vi "vibrate_and_record.vi"(3 "SSH password":string, 4 "Transfer and Run Date Folder After Experiment":bool, 5 "SSH user name":string, 6 "Tags":string, 7 "Frames":i32, 8 "frequencies":dbl[](array[numeric]), 9 "PWM duty cycles":dbl[](array[numeric]), 10 "parameters":string[](array[string]), 11 "parameters headers":string[](array[string])) -> ()   [LabVIEW 2014]
uses:
  <vilib>/userdefined/High Color/IMAQdx.ctl
  <vilib>/Utility/file.llb/Write To Spreadsheet File (DBL).vi
  <vilib>/Utility/file.llb/Write To Spreadsheet File (string).vi
  <vilib>/Utility/file.llb/Read From Spreadsheet File (string).vi
  <vilib>/vision/driver/NI_Vision_Acquisition_Software.lvlib
panel:
  out "Error":string
  out "Save Directory":path
  out "Buffer Number Out":u32
  out "Image":T1(plugin-control)
  in  "stop":bool
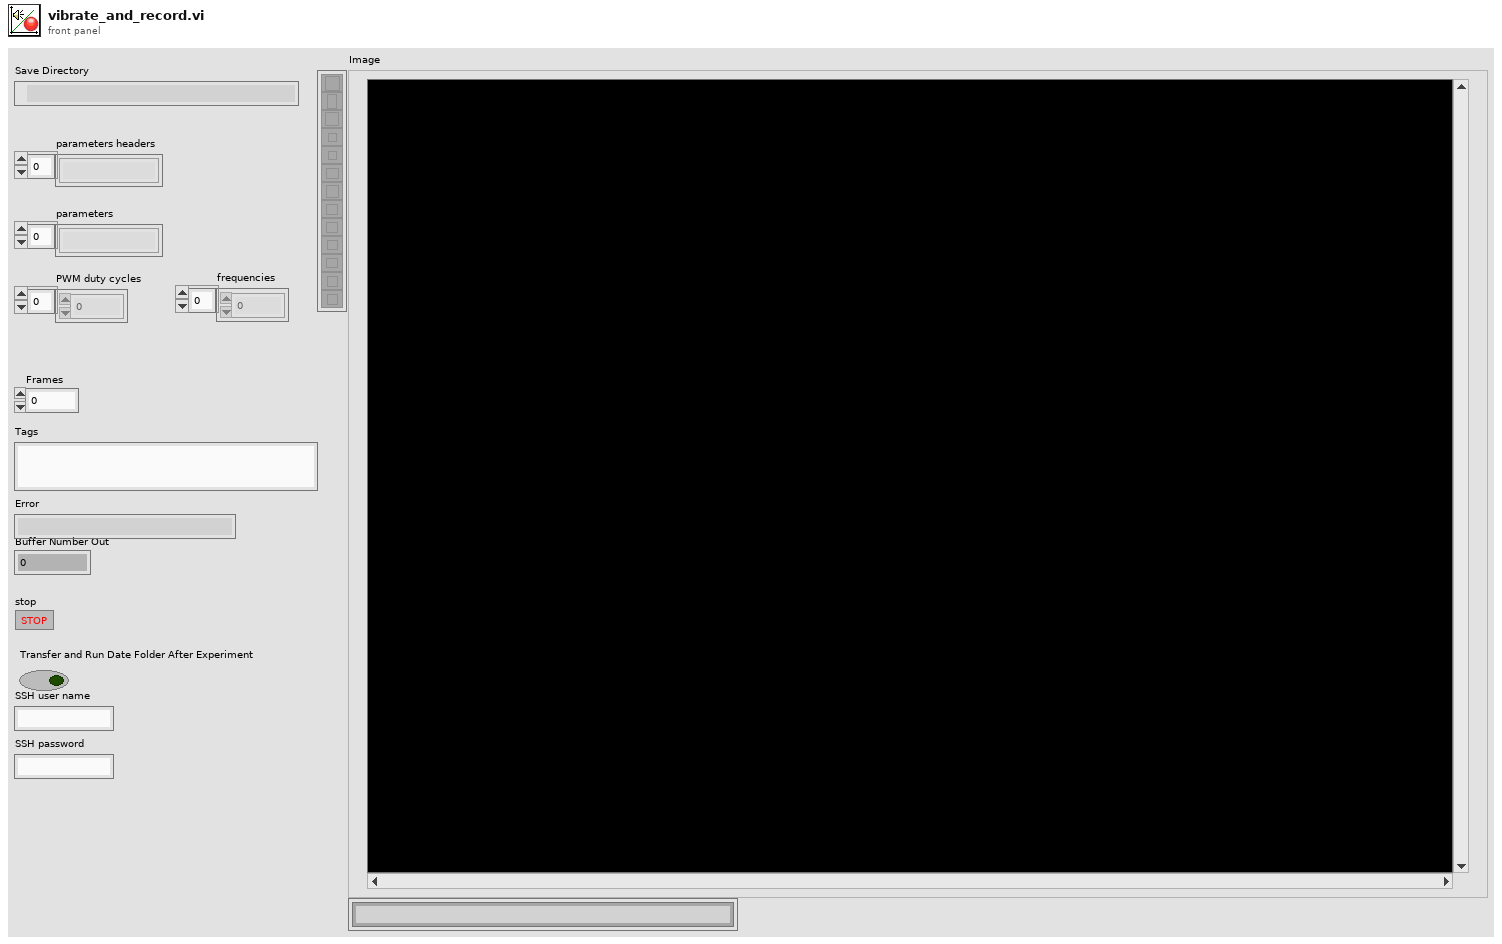
[diagram p1: front panel]
types:
  T1 = typedef "IMAQ Image.ctl" = refnum<image>
  T2 = typedef "IMAQdx.ctl" = refnum<k21>
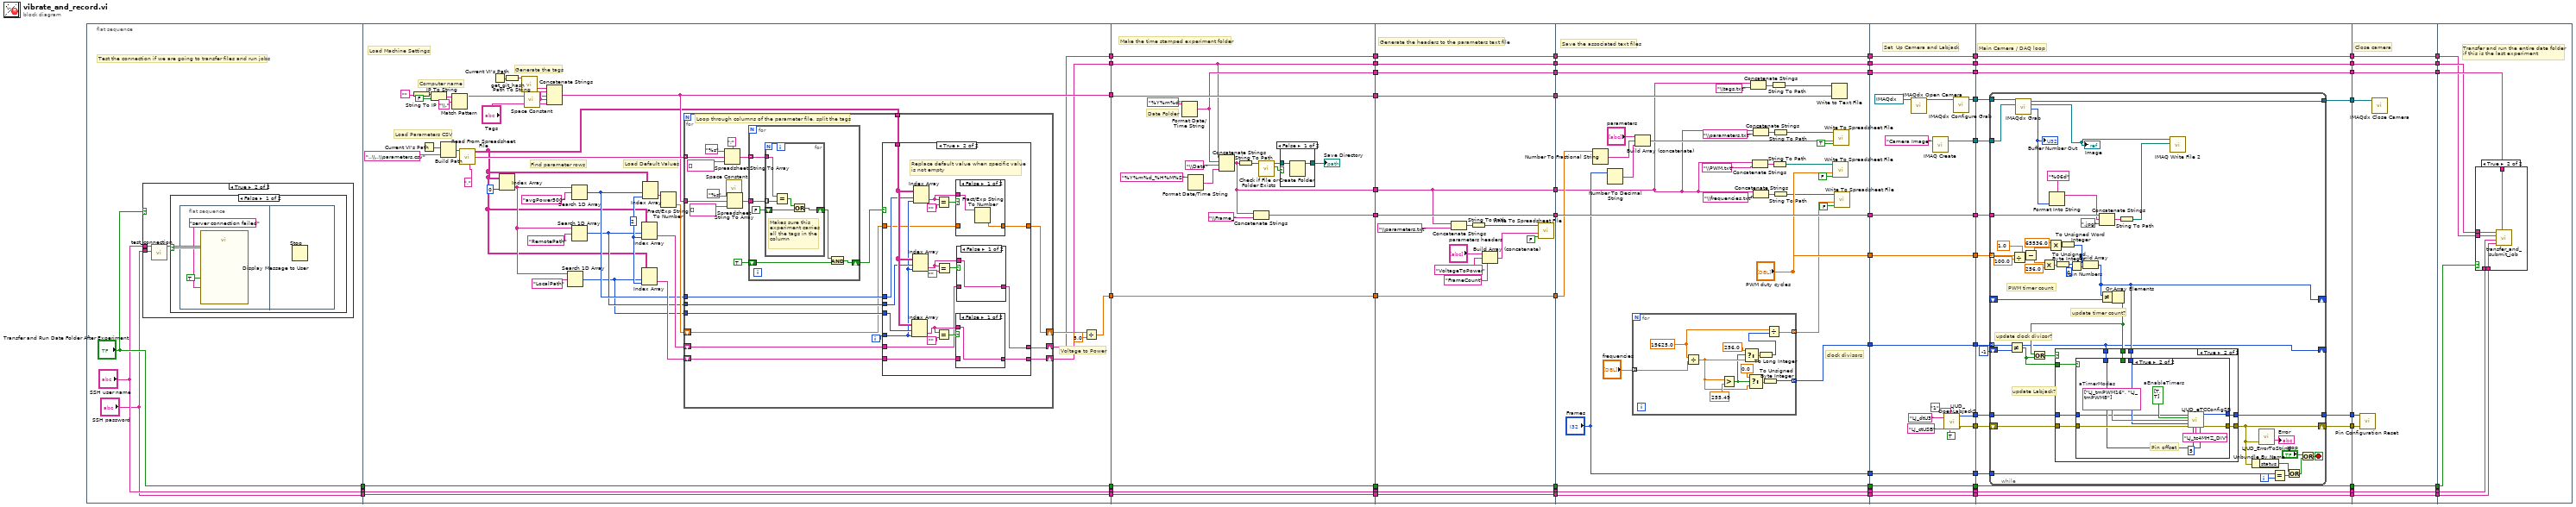
[diagram p0: block diagram]
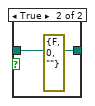
[diagram p8: hidden frame]
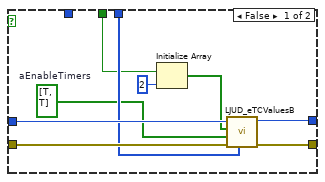
[diagram p10: hidden frame]
diagram:
  n1 = flat-sequence {
    tunnel: ["Transfer and Run Date Folder After Experiment"] -> w28
    tunnel: ["SSH user name"] -> w27
    tunnel: ["SSH password"] -> w26
    tunnel: [w108] -> w58
    tunnel: [w88] -> w57
    tunnel: [w78] -> w48
    tunnel: [w79] -> w47
    tunnel: w28 -> [w99]
    tunnel: w27 -> [w98]
    tunnel: w26 -> [w97]
    tunnel: [w99] -> w19
    tunnel: [w98] -> w12
    tunnel: [w97] -> w11
    tunnel: [w199] -> w42
    tunnel: [w198] -> w40
    tunnel: [w197] -> w38
    tunnel: [w196] -> w36
    tunnel: [w195] -> w34
    tunnel: [w194] -> w32
    tunnel: [w193] -> w30
    tunnel: w47 -> [w193]
    tunnel: w48 -> [w194]
    tunnel: w57 -> [w196]
    tunnel: w58 -> [w197]
    tunnel: [w183] -> w20
    tunnel: w19 -> [w183]
    tunnel: [w182] -> w13
    tunnel: w12 -> [w182]
    tunnel: w11 -> [w181]
    tunnel: [w181] -> w10
    tunnel: w42 -> [w220]
    tunnel: [w220] -> w41
    tunnel: w40 -> [w206]
    tunnel: [w206] -> w39
    tunnel: w38 -> [w219]
    tunnel: [w219] -> w37
    tunnel: w36 -> [w218]
    tunnel: [w218] -> w35
    tunnel: w34 -> [w217]
    tunnel: [w217] -> w33
    tunnel: w32 -> [w216]
    tunnel: [w216] -> w31
    tunnel: w30 -> [w215]
    tunnel: [w215] -> w29
    tunnel: [w205] -> w21
    tunnel: w20 -> [w205]
    tunnel: [w204] -> w14
    tunnel: w13 -> [w204]
    tunnel: w10 -> [w203]
    tunnel: [w203] -> w9
    tunnel: w41 -> [w252]
    tunnel: [w252] -> w63
    tunnel: ["PWM duty cycles"] -> w61
    tunnel: ["Frames"] -> w60
    tunnel: w39 -> [w224]
    tunnel: w37 -> [w235]
    tunnel: w35 -> [w230]
    tunnel: w33 -> [w241]
    tunnel: [w241] -> w53
    tunnel: [w240] -> w49
    tunnel: w31 -> [w240]
    tunnel: [w239] -> w43
    tunnel: w29 -> [w239]
    tunnel: [w233] -> w22
    tunnel: w21 -> [w233]
    tunnel: [w232] -> w15
    tunnel: w14 -> [w232]
    tunnel: w9 -> [w231]
    tunnel: [w231] -> w8
    tunnel: [w221] -> w4
    tunnel: w63 -> [w282]
    tunnel: [w284] -> w69
    tunnel: [w283] -> w68
    tunnel: [w282] -> w67
    tunnel: [w267] -> w65
    tunnel: [w268] -> w64
    tunnel: [w278] -> w62
    tunnel: w61 -> [w278]
    tunnel: w60 -> [w277]
    tunnel: [w277] -> w59
    tunnel: [w275] -> w54
    tunnel: w53 -> [w275]
    tunnel: [w274] -> w50
    tunnel: w49 -> [w274]
    tunnel: [w273] -> w44
    tunnel: w43 -> [w273]
    tunnel: [w272] -> w23
    tunnel: w22 -> [w272]
    tunnel: [w271] -> w16
    tunnel: w15 -> [w271]
    tunnel: w8 -> [w270]
    tunnel: [w270] -> w7
    tunnel: w4 -> [w269]
    tunnel: [w269] -> w3
    tunnel: w69 -> [w305]
    tunnel: w68 -> [w304]
    tunnel: w67 -> [w303]
    tunnel: [w302] -> w66
    tunnel: w65 -> [w301]
    tunnel: w64 -> [w300]
    tunnel: w62 -> [w299]
    tunnel: w59 -> [w298]
    tunnel: [w297] -> w55
    tunnel: w54 -> [w297]
    tunnel: [w296] -> w51
    tunnel: w50 -> [w296]
    tunnel: [w295] -> w45
    tunnel: w44 -> [w295]
    tunnel: [w294] -> w24
    tunnel: w23 -> [w294]
    tunnel: [w293] -> w17
    tunnel: w16 -> [w293]
    tunnel: w7 -> [w292]
    tunnel: [w292] -> w6
    tunnel: w3 -> [w289]
    tunnel: [w291] -> w2
    tunnel: [w290] -> w1
    tunnel: w66 -> [w387]
    tunnel: [w386] -> w56
    tunnel: w55 -> [w386]
    tunnel: [w385] -> w52
    tunnel: w51 -> [w385]
    tunnel: [w384] -> w46
    tunnel: w45 -> [w384]
    tunnel: [w383] -> w25
    tunnel: w24 -> [w383]
    tunnel: [w382] -> w18
    tunnel: w17 -> [w382]
    tunnel: w6 -> [w381]
    tunnel: [w381] -> w5
    tunnel: w2 -> [w380]
    tunnel: w1 -> [w379]
    tunnel: w56 -> [w393]
    tunnel: w52 -> [w392]
    tunnel: w46 -> [w391]
    tunnel: w25 -> [w390]
    tunnel: w18 -> [w389]
    tunnel: w5 -> [w388]
    frame #0 {
      # "Test the connection if we are going to transfer files and run jobs"
      n2 = case shown="True" "Transfer and Run Date Folder After Experiment" {
        tunnel: "SSH password" -> [_ w75]
        tunnel: "SSH user name" -> [_ w73]
        frame False {
        }
        frame True {
          n3 = call "test_connection.vi"("Username"=w73, "Password"=w75) -> ("Connection Successful"=w74:bool)  [unwired: 7 in]
          n4 = case shown="False" w74 {
            frame False {
              n5 = flat-sequence {
                frame #0 {
                  n6 = call "Display Message to User"("Enable"=TRUE, "Message"="server connection failed") -> ()  [unwired: 8 in, 2 out]
                }
                frame #1 {
                  n7 = Stop() -> ()  [unwired: 1 in]
                }
              }
            }
            frame True {
            }
          }
        }
      }
    }
    frame #1 {
      w90 = 2
      # "Generate the tags"
      # "Find parameter rows"
      # "Load Default Values"
      # "Voltage to Power"
      # "Load Parameters CSV"
      # "Computer name"
      # "Load Machine Settings"
      n8 = String To IP(1:"") -> (0:w116:u32)
      n9 = Current VI's Path() -> (path=w111:path)
      n10 = IP To String(1:FALSE, 2:w116) -> (0:w113:string)
      n11 = Build Path(base path=w111, name or relative path="..\\..\\parameters.csv") -> (appended path=w101:path)
      n12 = Match Pattern(string=w113, regular expression="\\.") -> (before substring=w91:string)  [unwired: 1 in, 3 out]
      n13 = call-poly <vilib>:"Read From Spreadsheet File.vi"("delimiter (\\t)"=",", "file path (dialog if empty)"=w101) -> ("first row"=w89:string[], "all rows"=w81:string[][])  [unwired: 5 in, 3 out]
      n14 = Current VI's Path() -> (path=w94:path)
      n15 = Index Array(array=w81, index (col)=0) -> (element=w102:string[])  [unwired: 1 in]
      n16 = Path To String(path=w94) -> (string=w93:string)
      n17 = call "get_git_hash.vi"("VI folder"=w93) -> ("github hash"=w96:string)  [unwired: 10 in]
      n18 = call <vilib>:"Space Constant.vi"() -> ("String"=w95:string)
      n19 = Concatenate Strings(w96, w95, w91, w95, "Tags") -> (w88:string)
      n20 = Search 1D Array(1D array=w102, element="LocalPath") -> (index of element=w82:i32)  [unwired: 1 in]
      n21 = Search 1D Array(1D array=w102, element="RemotePath") -> (index of element=w83:i32)  [unwired: 1 in]
      n22 = Search 1D Array(1D array=w102, element="avgPower500") -> (index of element=w84:i32)  [unwired: 1 in]
      n23 = Index Array(array=w81, index (row)=w83, index (col)=w90) -> (element=w86:string)
      n24 = Index Array(array=w81, index (row)=w82, index (col)=w90) -> (element=w85:string)
      n25 = Index Array(array=w81, index (row)=w84, index (col)=w90) -> (element=w104:string)
      n26 = Fract/Exp String To Number(string=w104) -> (number=w87:dbl)  [unwired: 3 in, 1 out]
      n27 = for {
        tunnel: w89 -> [w139] mode=indexing
        tunnel: w88 -> [w131]
        tunnel: w84 -> [w126]
        tunnel: w83 -> [w125]
        tunnel: w82 -> [w124]
        tunnel: w81 -> [w129]
        shift-right: [w121] -> w80
        shift-left: w87 -> [w122]
        shift-right: [w118] -> w79
        shift-left: w86 -> [w119]
        shift-right: [w117] -> w78
        shift-left: w85 -> [w120]
        i -> [w123]
        # "Loop through columns of the parameter file, split the tags"
        n28 = Spreadsheet String To Array(delimiter (Tab)=";", format string="%s", spreadsheet string=w139, array type (2D Dbl)=string[] []) -> (array=w135:string[])
        n29 = call <vilib>:"Space Constant.vi"() -> ("String"=w133:string)
        n30 = Spreadsheet String To Array(delimiter (Tab)=w133, format string="%s", spreadsheet string=w131, array type (2D Dbl)=string[] []) -> (array=w130:string[])
        n31 = for {
          tunnel: w135 -> [w175] mode=indexing
          tunnel: w130 -> [w174]
          shift-right: [w172] -> w127
          shift-left: TRUE -> [w170]
          n32 = for {
            tunnel: w175 -> [w180]
            tunnel: w174 -> [w179] mode=indexing
            shift-right: [w176] -> w171
            shift-left: FALSE -> [w177]
            # "Makes sure this\nexperiment carries\nall the tags in the\ncolumn"
            n33 = Equal?(x=w180, y=w179) -> (x = y?=w178:bool)
            n34 = Or(x=w178, y=w177) -> (x .or. y?=w176:bool)
          }
          n35 = And(x=w171, y=w170) -> (x .and. y?=w172:bool)
        }
        n36 = case shown="True" w127 {
          tunnel: w122 -> [w142 w155]
          tunnel: [w142 w154] -> w121
          tunnel: w126 -> [_ w161]
          tunnel: w125 -> [_ w160]
          tunnel: w124 -> [_ w159]
          tunnel: w123 -> [_ w158]
          tunnel: w129 -> [_ w162]
          tunnel: [w141 w144] -> w118
          tunnel: [w140 w146] -> w117
          tunnel: w120 -> [w140 w145]
          tunnel: w119 -> [w141 w143]
          frame False {
          }
          frame True {
            # "Replace default value when specific value\nis not empty"
            n37 = Index Array(array=w162, index (row)=w159, index (col)=w158) -> (element=w147:string)
            n38 = Index Array(array=w162, index (row)=w160, index (col)=w158) -> (element=w150:string)
            n39 = Index Array(array=w162, index (row)=w161, index (col)=w158) -> (element=w153:string)
            n40 = Equal?(x=w153, y="") -> (x = y?=w156:bool)
            n41 = Equal?(x=w147, y="") -> (x = y?=w148:bool)
            n42 = Equal?(x=w150, y="") -> (x = y?=w151:bool)
            n43 = case shown="False" w156 {
              tunnel: w155 -> [_ w169]
              tunnel: [w168 w169] -> w154
              tunnel: w153 -> [w167 _]
              frame False {
                n44 = Fract/Exp String To Number(string=w167) -> (number=w168:dbl)  [unwired: 3 in, 1 out]
              }
              frame True {
              }
            }
            n45 = case shown="False" w148 {
              tunnel: w147 -> [w163 _]
              tunnel: [w163 w164] -> w146
              tunnel: w145 -> [_ w164]
              frame False {
              }
              frame True {
              }
            }
            n46 = case shown="False" w151 {
              tunnel: w150 -> [w165 _]
              tunnel: [w165 w166] -> w144
              tunnel: w143 -> [_ w166]
              frame False {
              }
              frame True {
              }
            }
          }
        }
      }
      n47 = Divide(x=w80, y=5.0) -> (x/y=w108:dbl)
    }
    frame #2 {
      # "Make the time stamped experiment folder"
      # "Date Folder"
      n48 = Format Date/Time String(time format string (%c)="%Y%m%d") -> (date/time string=w195:string)  [unwired: 2 in]
      n49 = Format Date/Time String(time format string (%c)="%Y%m%d_%H%M%S") -> (date/time string=w187:string)  [unwired: 2 in]
      n50 = Concatenate Strings(w194, w195, "\\Data", w187) -> (w198:string)
      n51 = String To Path(string=w198) -> (path=w186:path)
      n52 = Concatenate Strings(w198, "\\Frame_") -> (w199:string)
      n53 = call <vilib>:"Check if File or Folder Exists.vi"("path"=w186) -> ("file or folder exists?"=w191:bool, "dup path"=w190:path)  [unwired: 8 in, 1 out]
      n54 = case shown="False" w191 {
        tunnel: [w200 w202] -> w185
        tunnel: w190 -> [w201 w202]
        frame False {
          n55 = Create Folder(path (use dialog)=w201) -> (created path=w200:path)  [unwired: 2 in, 2 out]
        }
        frame True {
          (unwired) errorcluster {"status"=FALSE, "code"=0, "source"=""} ("error out")
        }
      }
      "Save Directory" <- w185
    }
    frame #3 {
      # "Generate the headers to the parameters text file"
      n56 = Concatenate Strings(w206, "\\parameters.txt") -> (w214:string)
      n57 = String To Path(string=w214) -> (path=w213:path)
      n58 = Build Array (concatenate)("parameters headers", "VoltageToPower", "FrameCount") -> (w210:string[])
      n59 = call-poly <vilib>:"Write To Spreadsheet File.vi"("append to file? (new file:F)"=FALSE, "1D data"=w210, "file path (dialog if empty)"=w213) -> ()  [unwired: 5 in, 1 out]
    }
    frame #4 {
      # "clock divisors"
      # "Save the associated text files"
      n60 = Number To Fractional String(number=w235) -> (F-format string=w236:string)  [unwired: 3 in]
      n61 = Number To Decimal String(number="Frames") -> (decimal integer string=w237:string)  [unwired: 1 in]
      n62 = for {
        tunnel: [w258] -> w222 mode=indexing
        tunnel: [w257] -> w221 mode=indexing
        tunnel: "frequencies" -> [w256] mode=indexing
        w255 = 15625.0 ("x")
        n63 = Divide(x=w255, y=w256) -> (x/y=w261:dbl)
        n64 = Greater?(x=w261, y=255.49) -> (0:w260:bool)
        n65 = Select(t=256.0, s=w260, f=w261) -> (s? t:f=w263:dbl)
        n66 = Select(t=0.0, s=w260, f=w261) -> (s? t:f=w264:dbl)
        n67 = To Long Integer(number=w263) -> (32bit integer=w259:i32)
        n68 = To Unsigned Byte Integer(number=w264) -> (unsigned 8bit integer=w257:u8)
        n69 = Divide(x=w255, y=w259) -> (x/y=w258:dbl)
      }
      n70 = Build Array (concatenate)("parameters", w236, w237) -> (w245:string[])
      n71 = Concatenate Strings(w224, "\\tags.txt") -> (w243:string)
      n72 = Concatenate Strings(w224, "\\PWM.txt") -> (w254:string)
      n73 = Concatenate Strings(w224, "\\parameters.txt") -> (w249:string)
      n74 = Concatenate Strings(w224, "\\frequencies.txt") -> (w228:string)
      n75 = String To Path(string=w243) -> (path=w242:path)
      n76 = String To Path(string=w254) -> (path=w253:path)
      n77 = String To Path(string=w249) -> (path=w248:path)
      n78 = String To Path(string=w228) -> (path=w227:path)
      n79 = Write to Text File(file (use dialog)=w242, text=w230) -> ()  [unwired: 2 in, 3 out]
      n80 = call-poly <vilib>:"Write To Spreadsheet File.vi"("append to file? (new file:F)"=FALSE, "1D data"="PWM duty cycles", "file path (dialog if empty)"=w253) -> ()  [unwired: 5 in, 1 out]
      n81 = call-poly <vilib>:"Write To Spreadsheet File.vi"("append to file? (new file:F)"=TRUE, "1D data"=w245, "file path (dialog if empty)"=w248) -> ()  [unwired: 5 in, 1 out]
      n82 = call-poly <vilib>:"Write To Spreadsheet File.vi"("append to file? (new file:F)"=FALSE, "1D data"=w222, "file path (dialog if empty)"=w227) -> ()  [unwired: 5 in, 1 out]
    }
    frame #5 {
      # "Set  Up Camera and Labjack"
      n83 = call <vilib>:"IMAQdx Open Camera.vi"("Session In"=T2 "cam0") -> ("Session Out"=w286:T2)  [unwired: 9 in, 1 out]
      n84 = call "IMAQ Create"("Image Name"="Camera Image") -> ("New Image"=w283:T1)  [unwired: 4 in, 1 out]
      n85 = call "LJUD_OpenLabJackS.vi"("FirstFound"=TRUE, "Address"="1" ("DeviceType"), "ConnectionType"="LJ_ctUSB", "DeviceType"="LJ_dtU3") -> ("error out"=w268:errorcluster, "Handle"=w267:i32)  [unwired: 5 in, 1 out]
      n86 = call <vilib>:"IMAQdx Configure Grab.vi"("Session In"=w286) -> ("Session Out"=w284:T2)  [unwired: 9 in, 1 out]
    }
    frame #6 {
      # "Main Camera / DAQ loop"
      n87 = while {
        tunnel: w305 -> [w349]
        tunnel: [w348] -> w302
        tunnel: w304 -> [w347]
        tunnel: w303 -> [w345]
        tunnel: w301 -> [w318]
        shift-right: [w311] -> w291
        shift-left: w300 -> [w316]
        tunnel: w299 -> [w326] mode=indexing
        tunnel: w298 -> [w312]
        tunnel: [w317] -> w290
        shift-right: [w310] -> _
        shift-left: _ -> [w322]
        tunnel: w289 -> [w308] mode=indexing
        shift-right: [w308] -> _
        shift-left: -1 -> [w321]
        i -> [w315]
        stop <- w338 stop-if-true
        # "update timer count?"
        # "update Labjack?"
        # "update clock divisor?"
        # "PWM timer count"
        n88 = Not Equal?(x=w308, y=w321) -> (x != y?=w319:bool)
        n89 = Divide(x=w326, y=100.0) -> (x/y=w333:dbl)
        n90 = call <vilib>:"IMAQdx Grab.vi"("Image In"=w347, "Session In"=w349) -> ("Buffer Number Out"=w341:u32, "Image Out"=w346:T1, "Session Out"=w348:T2)  [unwired: 6 in, 1 out]
        "Image" <- w346
        "Buffer Number Out" <- w341
        n91 = Subtract(x=1.0, y=w333) -> (x-y=w324:dbl)
        n92 = Multiply(x=w324, y=256.0) -> (x*y=w335:dbl)
        n93 = Multiply(x=65536.0 ("y"), y=w324) -> (x*y=w331:dbl)
        n94 = Format Into String(format string="%06d" ("string"), w341) -> (resulting string=w340:string)  [unwired: 2 in, 1 out]
        n95 = To Unsigned Byte Integer(number=w335) -> (unsigned 8bit integer=w328:u8)
        n96 = To Unsigned Word Integer(number=w331) -> (unsigned 16bit integer=w330:u16)
        n97 = Join Numbers(hi=w328, lo=u8 0) -> ((hi.lo)=w329:u16)
        n98 = Build Array(w330, w329) -> (w310:u16[])
        n99 = Concatenate Strings(w345, w340, ".jpg" ("string")) -> (w343:string)
        n100 = Not Equal?(x=w310, y=w322) -> (x != y?=w323:bool[])
        n101 = Or Array Elements(Boolean array=w323) -> (logical OR=w309:bool)
        n102 = Or(x=w309, y=w319) -> (x .or. y?=w320:bool)
        n103 = case shown="True" w320 {
          tunnel: w319 -> [_ w359]
          tunnel: w318 -> [w351 w358]
          tunnel: [w351 w357] -> w317
          tunnel: w316 -> [w350 w356]
          tunnel: [w350 w355] -> w311
          tunnel: w310 -> [_ w354]
          tunnel: w309 -> [_ w353]
          tunnel: w308 -> [_ w352]
          frame False {
          }
          frame True {
            n104 = case shown="True" w359 {
              tunnel: w358 -> [w365 w369]
              tunnel: [w367 w374] -> w357
              tunnel: w356 -> [w364 w373]
              tunnel: [w368 w372] -> w355
              tunnel: w354 -> [w362 w371]
              tunnel: w353 -> [w361 _]
              tunnel: w352 -> [_ w370]
              frame False {
                w360 = bool[] [TRUE, TRUE]  # aEnableTimers
                n105 = Initialize Array(w361, 2 ("Dimension Size")) -> (w363:bool[])
                n106 = call "LJUD_eTCValuesB.vi"("aTimerValues Write"=w362, "error in"=w364, "aUpdateResetTimers"=w360, "aReadTimers"=w363, "Handle In"=w365) -> ("error out"=w368:errorcluster, "Handle Out"=w367:i32)  [unwired: 3 in, 2 out]
              }
              frame True {
                w376 = bool[] [TRUE, TRUE]  # aEnableTimers
                w378 = string[] ["LJ_tmPWM16", "LJ_tmPWM8"]  # aTimerModes
                # "Pin offset"
                n107 = call "LJUD_eTCConfigSB.vi"("Handle In"=w369, "aEnableTimers"=w376, "aTimerModes"=w378, "aTimerValues"=w371, "error in"=w373, "TCPinOffset"=5, "TimerClockBase"="LJ_tc4MHZ_DIV" ("Timer Clock Base"), "TimerClockDivisor"=w370) -> ("Handle Out"=w374:i32, "error out"=w372:errorcluster)  [unwired: 6 in]
              }
            }
          }
        }
        n108 = String To Path(string=w343) -> (path=w342:path)
        n109 = call-poly "IMAQ Write File 2"("File Path"=w342, "Image"=w346) -> ()  [unwired: 8 in, 2 out]
        n110 = Unbundle By Name(w311) -> ("status"=w314:bool)
        n111 = call "LJUD_ErrorToString.vi"("error in"=w311) -> ("String"=→"Error":string)  [unwired: 10 in]
        n112 = Equal?(x=w312, y=w315) -> (x = y?=w313:bool)
        n113 = Or(x=w314, y=w313) -> (x .or. y?=w306:bool)
        n114 = Or(x="stop", y=w306) -> (x .or. y?=w338:bool)
      }
    }
    frame #7 {
      # "Close camera"
      n115 = call "Pin Configuration Reset.vi"("error in"=w380, "Handle In"=w379) -> ()  [unwired: 8 in, 2 out]
      n116 = call <vilib>:"IMAQdx Close Camera.vi"("Session In"=w387) -> ()  [unwired: 10 in, 1 out]
    }
    frame #8 {
      # "Transfer and run the entire date folder\nif this is the last experiment"
      n117 = case shown="True" w390 {
        tunnel: w393 -> [_ w398]
        tunnel: w392 -> [_ w397]
        tunnel: w391 -> [_ w396]
        tunnel: w389 -> [_ w395]
        tunnel: w388 -> [_ w394]
        frame False {
        }
        frame True {
          n118 = call "transfer_and_submit_job.vi"("Date Folder"=w398, "Password"=w394, "Username"=w395, "Remote Data Directory"=w396, "Local Data Directory"=w397) -> ()  [unwired: 7 in]
        }
      }
    }
  }
